vi "Assign Point Ramping IOP.vi"(4 "Accurus Ctrl Cluster":T1={"Stop Vacuum"=TRUE, "Vacuum Force"=0, "Max Limit [mmHg]"=600.0, "Slide in"=0, "Irrigation?"=TRUE} {"Slide in" scale=0.0..78.0; "Vacuum Force" min=0 max=78}, 5 "Ramp Time [sec]":dbl=3.0, 6 "L1 to L4 PID Cluster":T2={"L1 PID Gains"={"Kp"=0.005, "Kd"=0.5, "Ki"=0.0005}, "L2 PID Gains"={"Kp"=0.01, "Kd"=1.0, "Ki"=0.0005}, "L3 PID Gains"={"Kp"=0.05, "Kd"=1.0, "Ki"=0.0005}, "L4 PID Gains"={"Kp"=0.1, "Kd"=0.1, "Ki"=0.0005}}, 7 "Offset Home2RCM":dbl[](array[numeric])=[0.0, 0.0, 0.0, 0.0], 8 "Destination Posit Array [mm]":dbl[](array[numeric])=[0.0, 0.0, -3.0, 0.0], 9 "Previous Posit Array":dbl[](array[numeric])=[0.0, 0.0, 0.0, 0.0], 10 "error in":errorcluster, 11 "FPGA VI Reference In":refnum<k20>) -> (1 "Last L1 to L4 Posit":dbl[](array[numeric]), 2 "error out":errorcluster, 3 "FPGA VI Reference Out":refnum<k20>)   [LabVIEW 2016]
uses:
  <vilib>/Analysis/1siggen.llb/Ramp Pattern by Samples.vi
  Subsystems/Global Variables.vi
  <vilib>/Analysis/NI_AALBase.lvlib
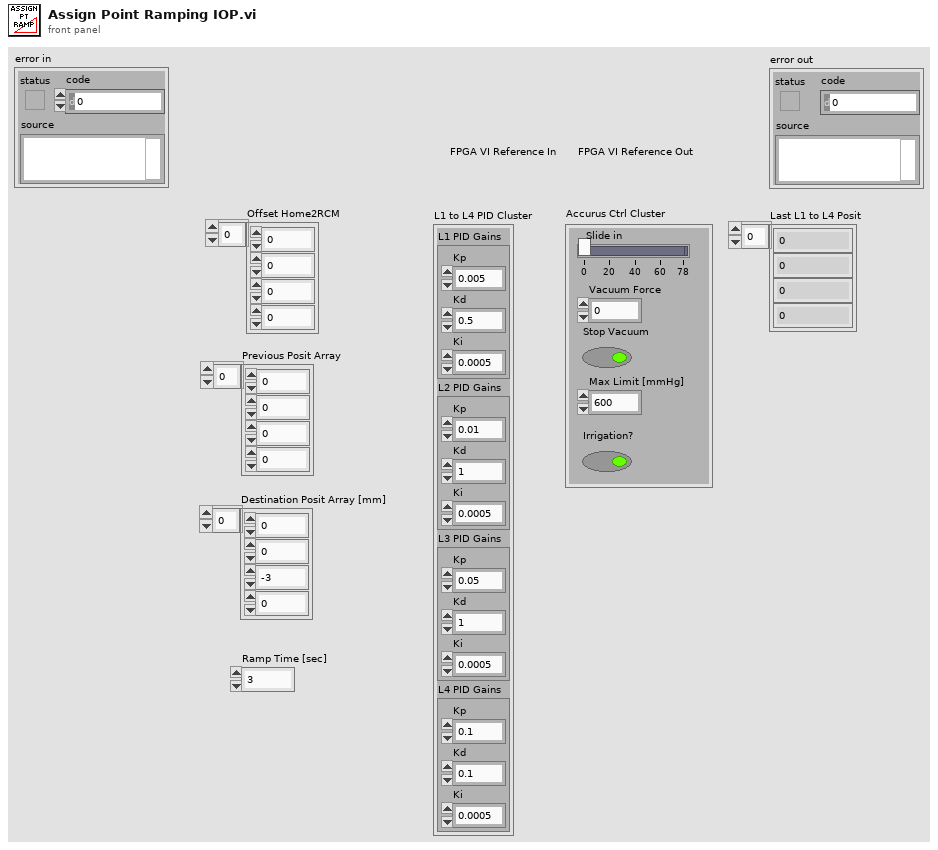
[diagram p1: front panel]
types:
  T1 = cluster{"Stop Vacuum":bool, "Vacuum Force":i8, "Max Limit [mmHg]":dbl, "Slide in":i8, "Irrigation?":bool}
  T2 = cluster{"L1 PID Gains":cluster{"Kp":dbl, "Kd":dbl, "Ki":dbl}, "L2 PID Gains":cluster{"Kp":dbl, "Kd":dbl, "Ki":dbl}, "L3 PID Gains":cluster{"Kp":dbl, "Kd":dbl, "Ki":dbl}, "L4 PID Gains":cluster{"Kp":dbl, "Kd":dbl, "Ki":dbl}}
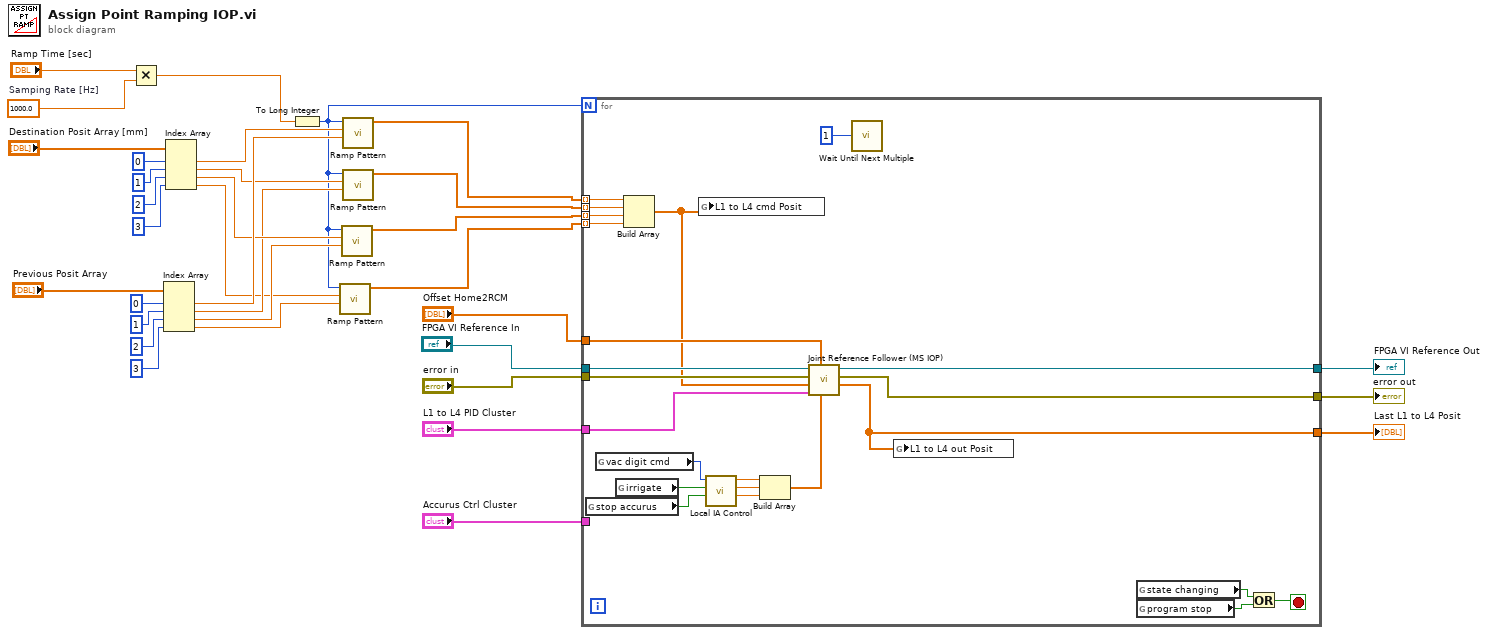
[diagram p0: block diagram]
diagram:
  w23 = 1000.0  # Samping Rate [Hz]
  n1 = Multiply(x="Ramp Time [sec]", y=w23) -> (x*y=w14:dbl)
  n2 = Index Array(array="Previous Posit Array", index #1=0 ("index"), index #2=1 ("index"), index #3=2 ("index"), index #4=3 ("index")) -> (element #1=w22:dbl, element #2=w18:dbl, element #3=w17:dbl, element #4=w16:dbl)
  n3 = Index Array(array="Destination Posit Array [mm]", index #1=0 ("index"), index #2=1 ("index"), index #3=2 ("index"), index #4=3 ("index")) -> (element #1=w21:dbl, element #2=w20:dbl, element #3=w19:dbl, element #4=w15:dbl)
  n4 = To Long Integer(number=w14) -> (32bit integer=w13:i32)
  n5 = call-poly <vilib>:"Ramp Pattern.vi"("start"=w16, "end"=w15, "samples"=w13) -> ("Ramp Pattern"=w9:dbl[])  [unwired: 7 in, 1 out]
  n6 = call-poly <vilib>:"Ramp Pattern.vi"("start"=w17, "end"=w19, "samples"=w13) -> ("Ramp Pattern"=w10:dbl[])  [unwired: 7 in, 1 out]
  n7 = call-poly <vilib>:"Ramp Pattern.vi"("start"=w22, "end"=w21, "samples"=w13) -> ("Ramp Pattern"=w12:dbl[])  [unwired: 7 in, 1 out]
  n8 = call-poly <vilib>:"Ramp Pattern.vi"("start"=w18, "end"=w20, "samples"=w13) -> ("Ramp Pattern"=w11:dbl[])  [unwired: 7 in, 1 out]
  n9 = for {
    N: w13 -> [_]
    tunnel: w12 -> [w57] mode=indexing
    tunnel: w11 -> [w56] mode=indexing
    tunnel: w10 -> [w55] mode=indexing
    tunnel: w9 -> [w54] mode=indexing
    tunnel: [w48] -> w1
    tunnel: [w42] -> w5
    tunnel: "Offset Home2RCM" -> [w49]
    tunnel: "L1 to L4 PID Cluster" -> [w44]
    tunnel: [w43] -> w7
    tunnel: "FPGA VI Reference In" -> [w47]
    tunnel: "error in" -> [w46]
    tunnel: "Accurus Ctrl Cluster" -> [_]
    stop <- w50 stop-if-true
    n10 = global read "Global Variables.vi" "stop accurus"() -> (w38:bool)
    n11 = global read "Global Variables.vi" "vac digit cmd"() -> (w35:i8)
    n12 = global read "Global Variables.vi" "irrigate"() -> (w37:bool)
    n13 = Build Array(w57, w56, w55, w54) -> (w45:dbl[])
    n14 = global write "Global Variables.vi" "L1 to L4 cmd Posit"(w45) -> ()
    n15 = call "Local IA Control.vi"("E-Stop Vacuum"=w38, "Irrigate?"=w37, "8bit integer"=w35) -> ("Accurus Engaged Vout"=w41:dbl, "Accurus ChB Vout"=w40:dbl, "Accurus ChA Vout"=w39:dbl)  [unwired: 6 in]
    n16 = Build Array(w39, w40, w41) -> (w36:dbl[])
    n17 = call "Joint Reference Follower (MS IOP).vi"("Acc Ctrl Array"=w36, "Offset Home2RCM [deg/mm]"=w49, "PID Ctrl Cluster"=w44, "Ref Array [deg/mm]"=w45, "error in"=w46, "FPGA VI Reference In"=w47) -> ("Output Posit Array [deg/mm]"=w43:dbl[], "error out"=w42:errorcluster, "FPGA VI Reference Out"=w48:refnum<k20>)  [unwired: 3 in]
    n18 = call "Wait Until Next Multiple"("Count(mSec)"=u32 1) -> ()  [unwired: 1 out]
    n19 = global write "Global Variables.vi" "L1 to L4 out Posit"(w43) -> ()
    n20 = global read "Global Variables.vi" "state changing"() -> (w52:bool)
    n21 = global read "Global Variables.vi" "program stop"() -> (w51:bool)
    n22 = Or(x=w52, y=w51) -> (x .or. y?=w50:bool)
  }
  "error out" <- w5
  "Last L1 to L4 Posit" <- w7
  "FPGA VI Reference Out" <- w1
